vi "Remove Termination Character.vi"(9 "Input string":string) -> (1 "String before CR+LF":string)   [LabVIEW 2018, in "Olympus IX BX Series.lvlib"]
doc: "This VI remove last new line characters."
uses:
  Olympus IX BX Series.lvlib
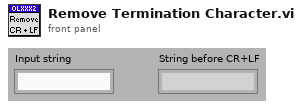
[diagram p1: front panel]
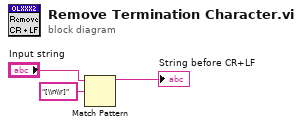
[diagram p0: block diagram]
diagram:
  n1 = Match Pattern(string="Input string", regular expression="[\\n\\r]") -> (before substring=→"String before CR+LF":string)  [unwired: 1 in, 3 out]
